vi "Tick Coordinate.vi"(2 "Direction":T2, 3 "Coordinate":T1) -> (1 "Coordinate Out":T1)   [LabVIEW 2019]
uses:
  Coordinate STYP.ctl
  Direction STYP.ctl
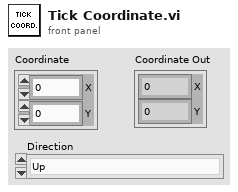
[diagram p1: front panel]
types:
  T1 = typedef "Coordinate STYP.ctl" = cluster{"X":i32, "Y":i32}
  T2 = typedef "Direction STYP.ctl" = enum16{"Up", "Down", "Left", "Right"}
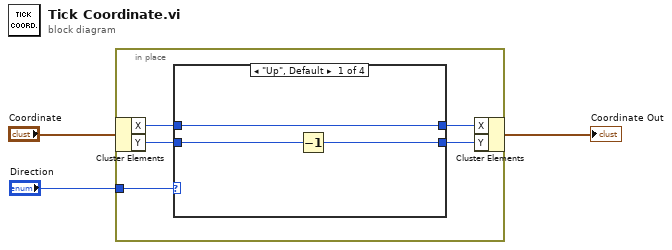
[diagram p0: block diagram]
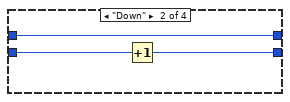
[diagram p2: hidden frame]
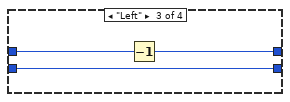
[diagram p3: hidden frame]
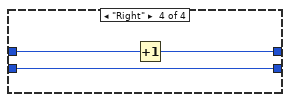
[diagram p4: hidden frame]
diagram:
  n1 = in-place {
    in-place-border: "Direction" -> [w4]
    n2 = in-place-cluster #1("Coordinate") -> ("X"=w8:i32, "Y"=w7:i32)
    n3 = case shown="\"Up\", Default" w4 {
      tunnel: w8 -> [w11 w14 w17 w20]
      tunnel: w7 -> [w10 w13 w16 w19]
      tunnel: [w11 w14 w15 w18] -> w6
      tunnel: [w9 w12 w16 w19] -> w5
      frame "Up", Default {
        n4 = Decrement(x=w10) -> (x-1=w9:i32)
      }
      frame "Down" {
        n5 = Increment(x=w13) -> (x+1=w12:i32)
      }
      frame "Left" {
        n6 = Decrement(x=w17) -> (x-1=w15:i32)
      }
      frame "Right" {
        n7 = Increment(x=w20) -> (x+1=w18:i32)
      }
    }
    n8 = in-place-cluster #1("X"=w6, "Y"=w5) -> (→"Coordinate Out":T1)
  }
